vi "TR_UNIT_ARR_2_STR_ARR.vi"(1 "offset":i32, 7 "TR_Unit_Arr":T1[](array[typedef]), 12 "format":enum16{"hex", "dec", "oct", "bin"}(ring), 13 "ForceString":bool, 14 "TSFormat":enum16{"原始值", "实际值"}(ring)) -> (3 "smb":i32[](array[numeric]), 8 "strTable":string[][](array[string]))   [LabVIEW 2011]
uses:
  _USB_CAN_T_R_Unit_.ctl
  _USB_CAN_GLOBAL_.vi
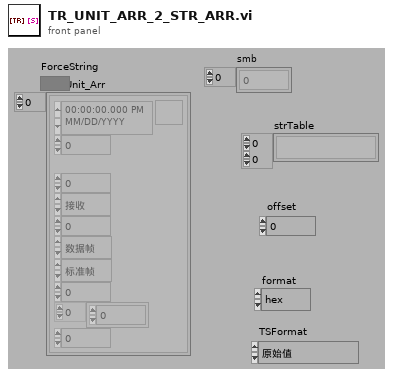
[diagram p1: front panel]
types:
  T1 = typedef "_USB_CAN_T_R_Unit_.ctl" = cluster{"time":timestamp, "channel":u16, "TimeStamp":u32, "tr":enum16{"接收", "发送"}, "id":u32, "Type":enum16{"数据帧", "远程帧"}, "Format":enum16{"标准帧", "扩展帧"}, "len":u8, "data":u8[], "sysTime":u32}
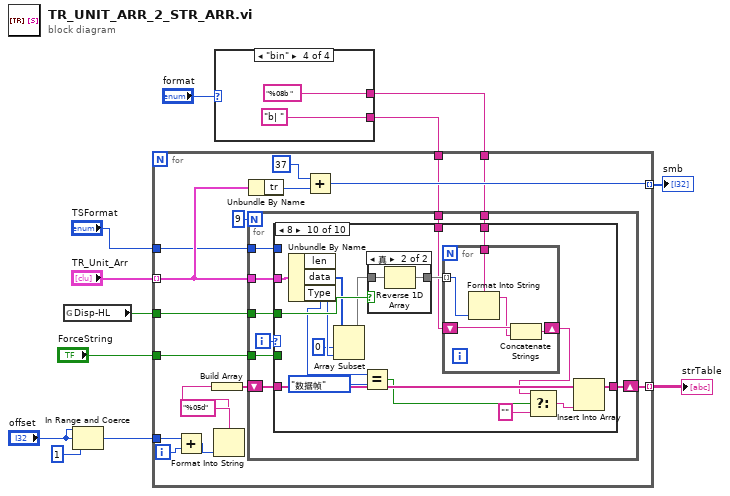
[diagram p0: block diagram]
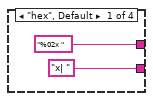
[diagram p2: hidden frame]
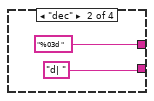
[diagram p3: hidden frame]
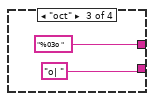
[diagram p4: hidden frame]
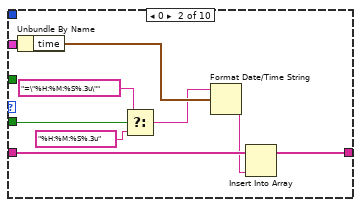
[diagram p6: hidden frame]
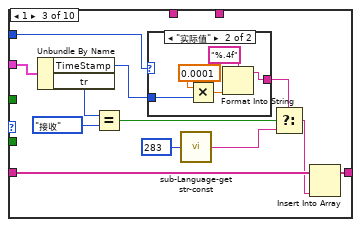
[diagram p7: hidden frame]
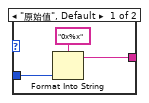
[diagram p8: hidden frame]
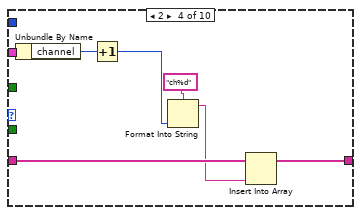
[diagram p9: hidden frame]
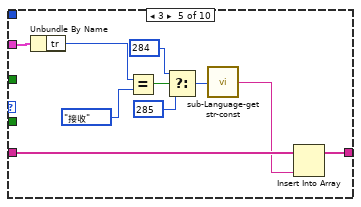
[diagram p10: hidden frame]
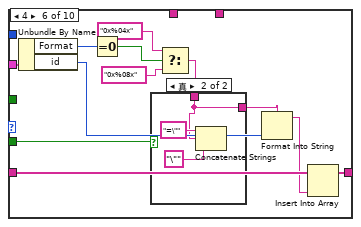
[diagram p11: hidden frame]
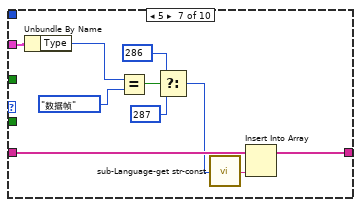
[diagram p13: hidden frame]
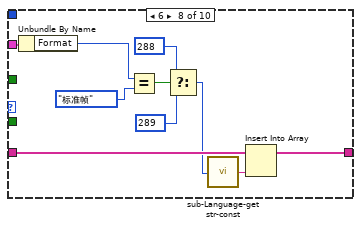
[diagram p14: hidden frame]
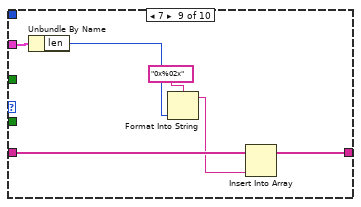
[diagram p15: hidden frame]
diagram:
  n1 = global read "_USB_CAN_GLOBAL_.vi" "Disp-HL"() -> (w9:bool)
  n2 = In Range and Coerce(upper limit="offset", x="offset", lower limit=1 ("下限")) -> (coerced(x)=w5:i32)  [unwired: 1 out]
  n3 = case shown="\"bin\"" "format" {
    tunnel: ["%02x " ("格式字符串") "%03d " ("格式字符串") "%03o " ("格式字符串") "%08b " ("格式字符串")] -> w7
    tunnel: ["x| " ("格式字符串") "d| " ("格式字符串") "o| " ("格式字符串") "b| " ("格式字符串")] -> w6
    frame "hex", Default {
    }
    frame "dec" {
    }
    frame "oct" {
    }
    frame "bin" {
    }
  }
  n4 = for {
    tunnel: "TR_Unit_Arr" -> [w29] mode=indexing
    tunnel: [w33] -> w12 mode=indexing
    tunnel: w5 -> [w31]
    tunnel: [w26] -> w10 mode=indexing
    tunnel: w9 -> [w25]
    tunnel: w7 -> [w24]
    tunnel: w6 -> [w23]
    tunnel: "TSFormat" -> [w22]
    tunnel: "ForceString" -> [w21]
    i -> [w32]
    n5 = Add(x=w31, y=w32) -> (x+y=w30:i32)
    n6 = Format Into String(format string="%05d" ("格式字符串"), w30) -> (resulting string=w36:string)  [unwired: 2 in, 1 out]
    n7 = Build Array(w36) -> (w35:string[])
    n8 = for {
      N: 9 -> [_]
      shift-right: [w43] -> w33
      shift-left: w35 -> [w45]
      tunnel: w29 -> [w44]
      tunnel: w25 -> [w42]
      tunnel: w24 -> [w41]
      tunnel: w23 -> [w40]
      tunnel: w22 -> [w39]
      tunnel: w21 -> [w38]
      i -> [w46]
      n9 = case shown="8" w46 {
        tunnel: w45 -> [w47 w54 w67 w82 w92 w104 w118 w128 w134 w151]
        tunnel: w44 -> [_ w56 w68 w83 w93 w105 w119 w129 w135 w152]
        tunnel: [w47 w52 w66 w81 w91 w103 w117 w127 w133 w150] -> w43
        tunnel: w42 -> [_ _ _ _ _ _ _ _ _ w148]
        tunnel: w41 -> [_ _ _ _ _ _ _ _ _ w147]
        tunnel: w40 -> [_ _ _ _ _ _ _ _ _ w146]
        tunnel: w39 -> [_ _ w59 _ _ _ _ _ _ _]
        tunnel: w38 -> [_ w50 _ _ _ w96 _ _ _ _]
        frame -1, Default {
        }
        frame 0 {
          n10 = Unbundle By Name(w56) -> ("time"=w55:timestamp)
          n11 = Select(t="=\"%H:%M:%S%.3u\"" ("时间格式字符串(%c)"), s=w50, f="%H:%M:%S%.3u" ("时间格式字符串(%c)")) -> (s? t:f=w48:string)
          n12 = Format Date/Time String(time format string (%c)=w48, seconds (now)=w55) -> (date/time string=w53:string)  [unwired: 1 in]
          n13 = Insert Into Array(array=w54, new element=w53) -> (w52:string[])  [unwired: 1 in]
        }
        frame 1 {
          n14 = Unbundle By Name(w68) -> ("TimeStamp"=w62:u32, "tr"=w65:enum16{"接收", "发送"})
          n15 = Equal?(x=w65, y=enum16{"接收", "发送"}."接收") -> (x = y?=w63:bool)
          n16 = case shown="\"实际值\"" w59 {
            tunnel: w62 -> [w71 w76]
            tunnel: [w69 w72] -> w61
            frame "原始值", Default {
              n17 = Format Into String(format string="0x%x" ("格式字符串"), w71) -> (resulting string=w69:string)  [unwired: 2 in, 1 out]
            }
            frame "实际值" {
              n18 = Multiply(x=0.0001, y=w76) -> (x*y=w74:dbl)
              n19 = Format Into String(format string="%.4f" ("格式字符串"), w74) -> (resulting string=w72:string)  [unwired: 2 in, 1 out]
            }
          }
          n20 = call "sub-Language-get str-const.vi"("sid"=u32 283) -> ("str"=w57:string)
          n21 = Select(t=w61, s=w63, f=w57) -> (s? t:f=w60:string)
          n22 = Insert Into Array(array=w67, new element=w60) -> (w66:string[])  [unwired: 1 in]
        }
        frame 2 {
          n23 = Unbundle By Name(w83) -> ("channel"=w80:u16)
          n24 = Increment(x=w80) -> (x+1=w77:u16)
          n25 = Format Into String(format string="ch%d" ("格式字符串"), w77) -> (resulting string=w79:string)  [unwired: 2 in, 1 out]
          n26 = Insert Into Array(array=w82, new element=w79) -> (w81:string[])  [unwired: 1 in]
        }
        frame 3 {
          n27 = Unbundle By Name(w93) -> ("tr"=w89:enum16{"接收", "发送"})
          n28 = Equal?(x=w89, y=enum16{"接收", "发送"}."接收" ("tr")) -> (x = y?=w88:bool)
          n29 = Select(t=u32 284 ("sid"), s=w88, f=u32 285 ("sid")) -> (s? t:f=w85:u32)
          n30 = call "sub-Language-get str-const.vi"("sid"=w85) -> ("str"=w84:string)
          n31 = Insert Into Array(array=w92, new element=w84) -> (w91:string[])  [unwired: 1 in]
        }
        frame 4 {
          n32 = Unbundle By Name(w105) -> ("Format"=w100:enum16{"标准帧", "扩展帧"}, "id"=w102:u32)
          n33 = Equal To 0?(x=w100) -> (x = 0?=w99:bool)
          n34 = Select(t="0x%04x" ("格式字符串"), s=w99, f="0x%08x" ("格式字符串")) -> (s? t:f=w95:string)
          n35 = case shown="真" w96 {
            tunnel: w95 -> [w106 w107]
            tunnel: [w106 w107] -> w94
            frame False {
            }
            frame True {
              n36 = Concatenate Strings("=\"" ("字符串"), w107, "\"" ("字符串")) -> ()  [unwired: 1 out]
            }
          }
          n37 = Format Into String(format string=w94, w102) -> (resulting string=w101:string)  [unwired: 2 in, 1 out]
          n38 = Insert Into Array(array=w104, new element=w101) -> (w103:string[])  [unwired: 1 in]
        }
        frame 5 {
          n39 = Unbundle By Name(w119) -> ("Type"=w115:enum16{"数据帧", "远程帧"})
          n40 = Equal?(x=w115, y=enum16{"数据帧", "远程帧"}."数据帧" ("Type")) -> (x = y?=w116:bool)
          n41 = Select(t=u32 286 ("sid"), s=w116, f=u32 287 ("sid")) -> (s? t:f=w110:u32)
          n42 = call "sub-Language-get str-const.vi"("sid"=w110) -> ("str"=w111:string)
          n43 = Insert Into Array(array=w118, new element=w111) -> (w117:string[])  [unwired: 1 in]
        }
        frame 6 {
          n44 = Unbundle By Name(w129) -> ("Format"=w124:enum16{"标准帧", "扩展帧"})
          n45 = Equal?(x=w124, y=enum16{"标准帧", "扩展帧"}."标准帧" ("Format")) -> (x = y?=w126:bool)
          n46 = Select(t=u32 288 ("sid"), s=w126, f=u32 289 ("sid")) -> (s? t:f=w120:u32)
          n47 = call "sub-Language-get str-const.vi"("sid"=w120) -> ("str"=w121:string)
          n48 = Insert Into Array(array=w128, new element=w121) -> (w127:string[])  [unwired: 1 in]
        }
        frame 7 {
          n49 = Unbundle By Name(w135) -> ("len"=w132:u8)
          n50 = Format Into String(format string="0x%02x" ("格式字符串"), w132) -> (resulting string=w131:string)  [unwired: 2 in, 1 out]
          n51 = Insert Into Array(array=w134, new element=w131) -> (w133:string[])  [unwired: 1 in]
        }
        frame 8 {
          n52 = Unbundle By Name(w152) -> ("len"=w143:u8, "data"=w145:u8[], "Type"=w141:enum16{"数据帧", "远程帧"})
          n53 = Array Subset(array=w145, index=0 ("索引"), length=w143) -> (w144:u8[])
          n54 = Equal?(x=w141, y=enum16{"数据帧", "远程帧"}."数据帧") -> (x = y?=w139:bool)
          n55 = case shown="真" w148 {
            tunnel: w144 -> [w153 w155]
            tunnel: [w153 w154] -> w149
            frame False {
            }
            frame True {
              n56 = Reverse 1D Array(array=w155) -> (reversed array=w154:u8[])
            }
          }
          n57 = for {
            tunnel: w149 -> [w160] mode=indexing
            shift-right: [w159] -> w138
            shift-left: w146 -> [w158]
            tunnel: w147 -> [w156]
            n58 = Format Into String(format string=w156, w160) -> (resulting string=w157:string)  [unwired: 2 in, 1 out]
            n59 = Concatenate Strings(w158, w157) -> (w159:string)
          }
          n60 = Select(t=w138, s=w139, f="") -> (s? t:f=w136:string)
          n61 = Insert Into Array(array=w151, new element=w136) -> (w150:string[])  [unwired: 1 in]
        }
      }
    }
    n62 = Unbundle By Name(w29) -> ("tr"=w28:enum16{"接收", "发送"})
    n63 = Add(x=37, y=w28) -> (x+y=w26:i32)
  }
  "strTable" <- w12
  "smb" <- w10
